vi "Get Available Sets 1.0.vi"(8 "error in (no error)":errorcluster, 11 "Session in":refnum<k21>) -> (0 "error out":errorcluster, 2 "Software Sets":T1[](array[typedef]), 3 "Session out":refnum<k21>)   [LabVIEW 2017, in "nisyscfg.lvlib"]
uses:
  <vilib>/nisyscfg/nisyscfg.lvlib
  <vilib>/nisyscfg/Software Set.ctl
  <vilib>/nisyscfg/Software.ctl
  <vilib>/nisyscfg/Component Types.ctl
  <vilib>/nisyscfg/Get Available Sets.vi
panel:
  # "This cluster is deprecated.\nUse Software Set 1.2.ctl."
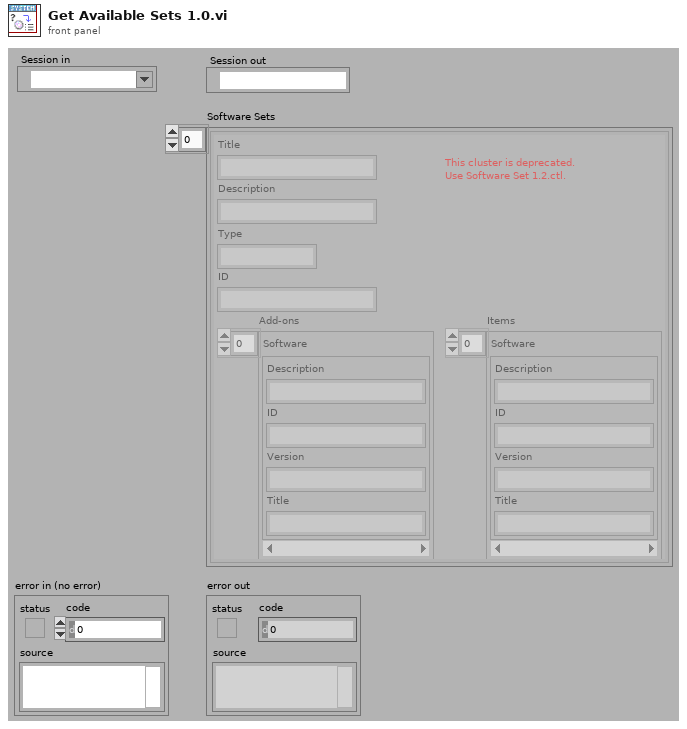
[diagram p1: front panel]
types:
  T1 = typedef "nisyscfg.lvlib/Software Set.ctl" = cluster{"Description":string, "ID":string, "Type":string, "Title":string, "Add-ons":T2[], "Items":T2[]}
  T2 = typedef "nisyscfg.lvlib/Software.ctl" = cluster{"Description":string, "ID":string, "Version":string, "Title":string}
  T3 = typedef "nisyscfg.lvlib/Component Types.ctl" = u32
  T4 = typedef "nisyscfg.lvlib/Software Set 1.2.ctl" = cluster{"information":T5, "items":T5[], "add-ons":T5[]}
  T5 = typedef "nisyscfg.lvlib/Software 1.2.ctl" = cluster{"title":string, "description":string, "ID":string, "version":string, "component type":T6}
  T6 = typedef "nisyscfg.lvlib/Component Type.ctl" = u32
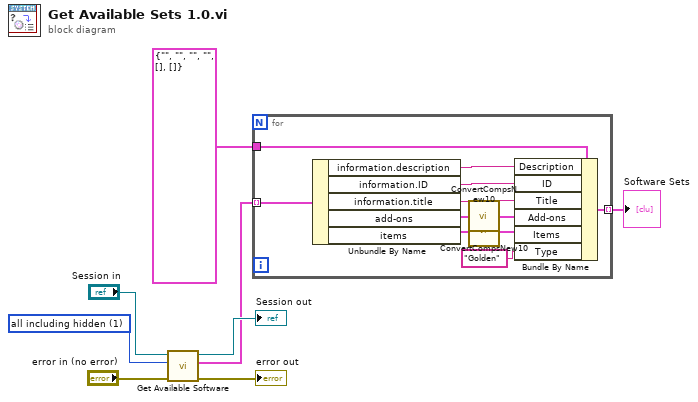
[diagram p0: block diagram]
diagram:
  w4 = T3 1 items=["all visible", "all including hidden"] ("item types (visible)")
  n1 = call-poly <vilib>:"Get Available Software.vi"("error in (no error)"="error in (no error)", "Item Types (all visible)"=w4, "Session in"="Session in") -> ("error out"=→"error out":errorcluster, "Software Sets"=w3:T4[], "Session out"=→"Session out":refnum<k21>)  [unwired: 6 in]
  n2 = for {
    tunnel: w3 -> [w19] mode=indexing
    tunnel: T1 {"Description"="", "ID"="", "Type"="", "Title"="", "Add-ons"=[], "Items"=[]} ("Software Set") -> [w18]
    tunnel: [w17] -> w1 mode=indexing
    n3 = Unbundle By Name(w19) -> ("information.description"=w9:string, "information.ID"=w10:string, "information.title"=w11:string, "add-ons"=w16:T5[], "items"=w15:T5[])
    n4 = call <vilib>:"ConvertCompsNew10.vi"("components 1.2"=w16) -> ("components 1.0"=w12:T2[])
    n5 = call <vilib>:"ConvertCompsNew10.vi"("components 1.2"=w15) -> ("components 1.0"=w13:T2[])
    n6 = Bundle By Name(cluster=w18, "Description"=w9, "ID"=w10, "Title"=w11, "Add-ons"=w12, "Items"=w13, "Type"="Golden") -> (w17:T1)
  }
  "Software Sets" <- w1
